vi "RobocadVMXTitan.vi"(8 "ErrorIn":errorcluster, 10 "InCluster":T4, 11 "Reference":T1) -> (0 "ErrorOut":errorcluster, 2 "OutCluster":T3, 3 "OutReference":T1)   [LabVIEW 2019]
uses:
  <vilib>/vision/Image Controls.llb/IMAQ Image.ctl
  C:/Users/user/Desktop/lvlib/assemblies/x86/LibraryForLabVIEW.dll
  assemblies/x86/LibraryForLabVIEW.dll
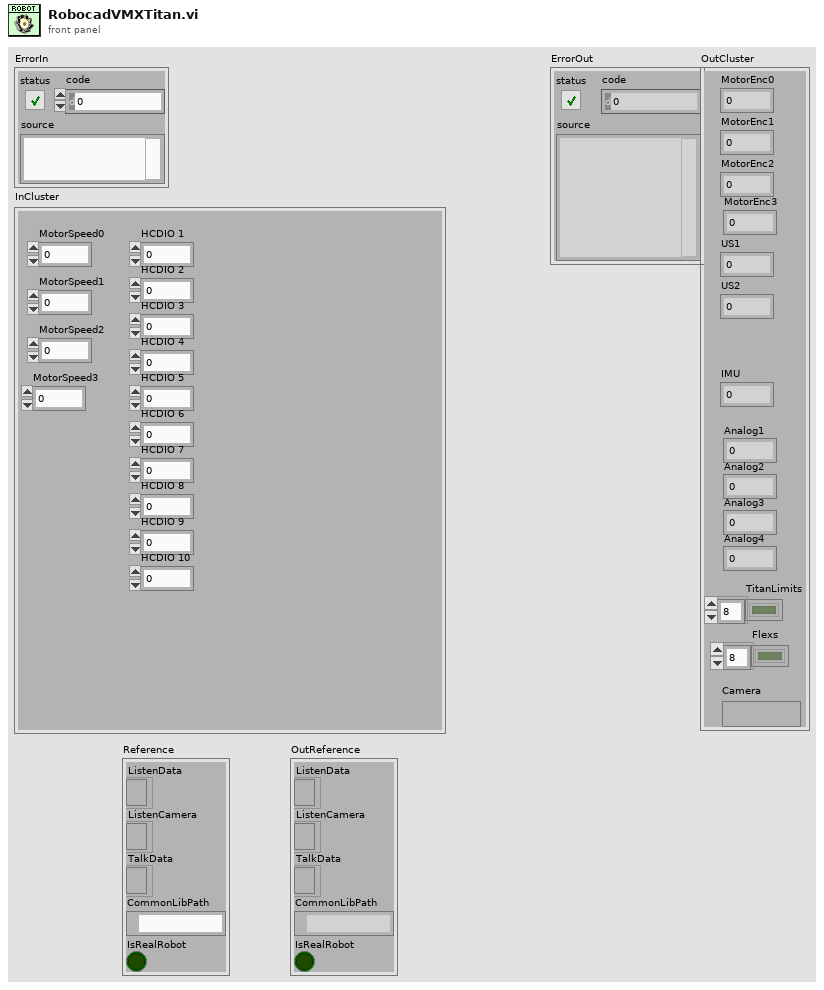
[diagram p1: front panel]
types:
  T1 = cluster{"ListenData":refnum<k24>, "ListenCamera":refnum<k24>, "TalkData":refnum<k24>, "CommonLibPath":path, "IsRealRobot":bool}
  T2 = typedef "IMAQ Image.ctl" = refnum<image>
  T3 = cluster{"MotorEnc0":dbl, "MotorEnc1":dbl, "MotorEnc2":dbl, "MotorEnc3":dbl, "US1":dbl, "US2":dbl, "Analog1":dbl, "Analog2":dbl, "Analog3":dbl, "Analog4":dbl, "IMU":dbl, "TitanLimits":bool[], "Flexs":bool[], "Camera":T2}
  T4 = cluster{"MotorSpeed0":dbl, "MotorSpeed1":dbl, "MotorSpeed2":dbl, "MotorSpeed3":dbl, "HCDIO 1":dbl, "HCDIO 2":dbl, "HCDIO 3":dbl, "HCDIO 4":dbl, "HCDIO 5":dbl, "HCDIO 6":dbl, "HCDIO 7":dbl, "HCDIO 8":dbl, "HCDIO 9":dbl, "HCDIO 10":dbl}
  T5 = cluster{"Encs":dbl[], "Sensors":dbl[], "TitanLimits":bool[], "Flexs":bool[], "Camera":T2}
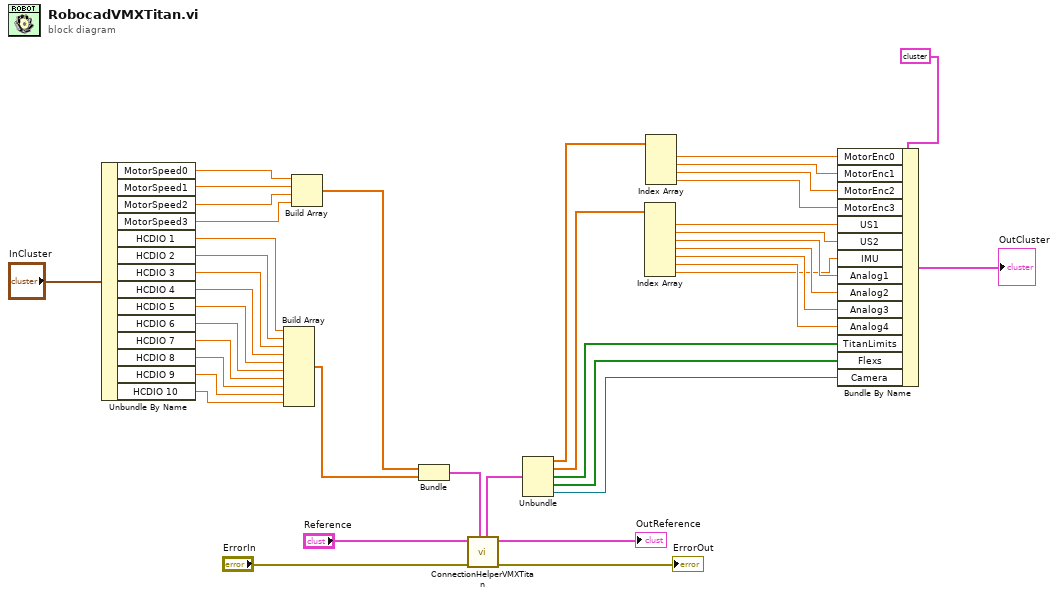
[diagram p0: block diagram]
diagram:
  n1 = Unbundle By Name("InCluster") -> ("MotorSpeed0"=w37:dbl, "MotorSpeed1"=w38:dbl, "MotorSpeed2"=w36:dbl, "MotorSpeed3"=w31:dbl, "HCDIO 1"=w26:dbl, "HCDIO 2"=w25:dbl, "HCDIO 3"=w24:dbl, "HCDIO 4"=w23:dbl, "HCDIO 5"=w22:dbl, "HCDIO 6"=w21:dbl, "HCDIO 7"=w20:dbl, "HCDIO 8"=w19:dbl, "HCDIO 9"=w18:dbl, "HCDIO 10"=w17:dbl)
  n2 = Build Array(w26, w25, w24, w23, w22, w21, w20, w19, w18, w17) -> (w27:dbl[])
  n3 = Build Array(w37, w38, w36, w31) -> (w35:dbl[])
  n4 = Bundle(w35, w27) -> (w16:cluster{dbl[], dbl[]})  [unwired: 1 in]
  n5 = call "ConnectionHelperVMXTitan.vi"("InCluster"=w16, "ErrorIn"="ErrorIn", "Reference"="Reference") -> ("ErrorOut"=→"ErrorOut":errorcluster, "OutReference"=→"OutReference":T1, "OutCluster"=w34:T5)  [unwired: 4 in]
  n6 = Unbundle(w34) -> ("Encs"=w33:dbl[], "Sensors"=w32:dbl[], "TitanLimits"=w7:bool[], "Flexs"=w6:bool[], "Camera"=w5:T2)
  n7 = Index Array(array=w32) -> (element #1=w14:dbl, element #2=w13:dbl, element #3=w12:dbl, element #4=w11:dbl, element #5=w10:dbl, element #6=w9:dbl, element #7=w8:dbl)  [unwired: 7 in]
  n8 = Index Array(array=w33) -> (element #1=w30:dbl, element #2=w29:dbl, element #3=w28:dbl, element #4=w15:dbl)  [unwired: 4 in]
  n9 = Bundle By Name(cluster=T3 {"MotorEnc0"=432600.0, "MotorEnc1"=-432600.0, "MotorEnc2"=0.0, "MotorEnc3"=96.69618, "US1"=96.45192, "US2"=90.32099, "Analog1"=0.0, "Analog2"=612.0, "Analog3"=612.0, "Analog4"=1310.0, "IMU"=1298.0, "TitanLimits"=[FALSE, FALSE, FALSE, FALSE, FALSE, FALSE, FALSE, FALSE], "Flexs"=[FALSE, FALSE, FALSE, FALSE, FALSE, FALSE, FALSE, FALSE], "Camera"="remote image 0000016AA53093F8"} ("OutCluster"), "MotorEnc0"=w30, "MotorEnc1"=w29, "MotorEnc2"=w28, "MotorEnc3"=w15, "US1"=w14, "US2"=w13, "IMU"=w8, "Analog1"=w12, "Analog2"=w11, "Analog3"=w10, "Analog4"=w9, "TitanLimits"=w7, "Flexs"=w6, "Camera"=w5) -> (→"OutCluster":T3)
